vi "ControllerMain.vi"(8 "Error In":errorcluster, 11 "Control Mode":T4(ring)) -> (0 "Error Out":errorcluster, 3 "Robot Inputs":T3, 4 "Joystick1DevRef":T1={"Device"=enum."USB 1"}, 5 "Stick0 Buttons":bool[](array[boolean]), 6 "Joystick0DevRef":T1={"Device"=enum."USB 1"}, 7 "Stick0 Axes":dbl[](array[numeric]))   [LabVIEW 2017]
uses:
  TeleopCommands.ctl
  <vilib>/Rock Robotics/WPI/Joystick/WPI_JoystickDevRef.ctl
  <vilib>/Rock Robotics/WPI/Joystick/WPI_JoystickDeviceEnum.ctl
  <vilib>/Rock Robotics/WPI/Utilities/WPI_GetSetVariantRefNum.vi
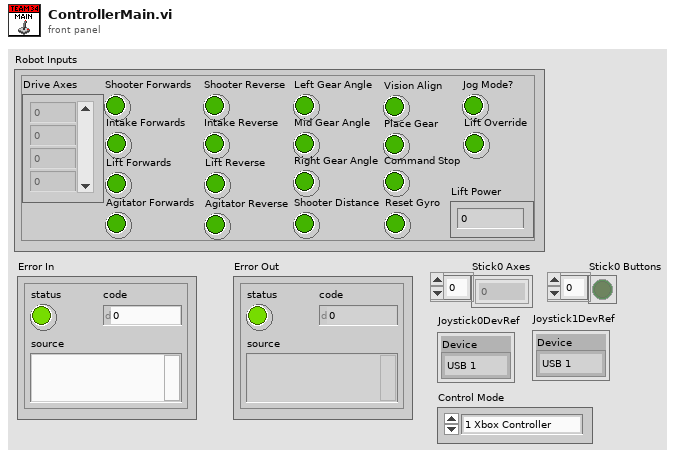
[diagram p1: front panel]
types:
  T1 = typedef "WPI_JoystickDevRef.ctl" = cluster{"Device":T2}
  T2 = typedef "WPI_JoystickDeviceEnum.ctl" = enum16{"USB 0", "USB 1", "USB 2", "USB 3", "USB 4", "USB 5"}
  T3 = typedef "TeleopCommands.ctl" = cluster{"Drive Axes":dbl[], "Shooter Forwards":bool, "Shooter Reverse":bool, "Intake Forwards":bool, "Intake Reverse":bool, "Lift Forwards":bool, "Lift Reverse":bool, "Agitator Forwards":bool, "Agitator Reverse":bool, "Left Gear Angle":bool, "Mid Gear Angle":bool, "Right Gear Angle":bool, "Shooter Distance":bool, "Vision Align":bool, "Place Gear":bool, "Command Stop":bool, "Reset Gyro":bool, "Jog Mode?":bool, "Lift Override":bool, "Lift Power":dbl}
  T4 = enum16{"1 Xbox Controller", "2 Xbox Controllers"}
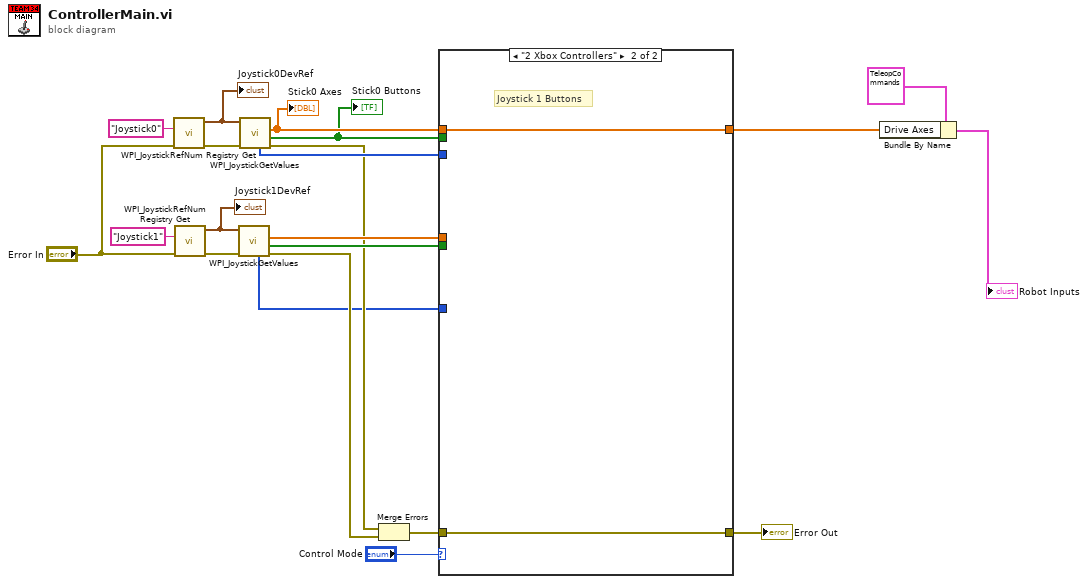
[diagram p0: block diagram]
diagram:
  n1 = call <vilib>:"WPI_JoystickRefNum Registry Get.vi"("error in (no error)"="Error In", "refnum name"="Joystick0") -> ("error out"=w16:errorcluster, "JoystickDevRef"=w21:T1)  [unwired: 8 out]
  "Joystick0DevRef" <- w21
  n2 = call <vilib>:"WPI_JoystickRefNum Registry Get.vi"("error in (no error)"="Error In", "refnum name"="Joystick1") -> ("error out"=w17:errorcluster, "JoystickDevRef"=w18:T1)  [unwired: 8 out]
  "Joystick1DevRef" <- w18
  n3 = call <vilib>:"WPI_JoystickGetValues.vi"("error in (no error)"=w17, "JoystickDevRef"=w18) -> ("error out"=w6:errorcluster, "Buttons"=w12:bool[], "Axes"=w11:dbl[], "POVs"=w3:i16[])  [unwired: 5 in, 1 out]
  n4 = call <vilib>:"WPI_JoystickGetValues.vi"("error in (no error)"=w16, "JoystickDevRef"=w21) -> ("error out"=w7:errorcluster, "Buttons"=w13:bool[], "Axes"=w14:dbl[], "POVs"=w9:i16[])  [unwired: 5 in, 1 out]
  "Stick0 Axes" <- w14
  "Stick0 Buttons" <- w13
  n5 = Merge Errors(w7, w6) -> (w5:errorcluster)
  n6 = case shown="\"2 Xbox Controllers\"" "Control Mode" {
    tunnel: w14 -> [w23 w25]
    tunnel: w13 -> [_ _]
    tunnel: w12 -> [_ _]
    tunnel: w11 -> [_ _]
    tunnel: [w23 w25] -> w10
    tunnel: w9 -> [_ _]
    tunnel: [w22 w24] -> w4
    tunnel: w5 -> [w22 w24]
    tunnel: w3 -> [_ _]
    frame "1 Xbox Controller", Default {
    }
    frame "2 Xbox Controllers" {
      # "Joystick 1 Buttons"
    }
  }
  "Error Out" <- w4
  n7 = Bundle By Name(cluster=T3 {"Drive Axes"=[], "Shooter Forwards"=FALSE, "Shooter Reverse"=FALSE, "Intake Forwards"=FALSE, "Intake Reverse"=FALSE, "Lift Forwards"=FALSE, "Lift Reverse"=FALSE, "Agitator Forwards"=FALSE, "Agitator Reverse"=FALSE, "Left Gear Angle"=FALSE, "Mid Gear Angle"=FALSE, "Right Gear Angle"=FALSE, "Shooter Distance"=FALSE, "Vision Align"=FALSE, "Place Gear"=FALSE, "Command Stop"=FALSE, "Reset Gyro"=FALSE, "Jog Mode?"=FALSE, "Lift Override"=FALSE, "Lift Power"=0.0} ("Robot Inputs"), "Drive Axes"=w10) -> (→"Robot Inputs":T3)
